vi "AutoDrive.vi"(9 "Target Robot Angle":dbl=-25.0, 10 "Distance":dbl=2000.0, 11 "Movement Angle":dbl) -> (1 "Done":bool=TRUE)   [LabVIEW 2017]
uses:
  Robot Global Data.vi
  <vilib>/addons/control/pid/pid.llb/PID (DBL).vi
  <vilib>/addons/control/pid/NI_PID_pid.lvlib
panel:
  in  "Allowable Encoder Error":dbl=425.0
  out "Encoder Out":dbl=1958.5
  out "output":dbl=0.037765 format="%.2f"
  out "output array":bool[](array[boolean])=[TRUE, TRUE, TRUE, TRUE, TRUE, TRUE, TRUE, TRUE, TRUE, TRUE]
  out "Encoder":cluster{"Robot Angle":dbl, "Gyro":dbl}(graph)={"Robot Angle"=0.0, "Gyro"=-25.0}
  in  "Encoder":dbl
  out "output - Distance":dbl(graph)=1958.5
  out "output - Angle":dbl(graph)=0.09727615381261338
  in  "PID gains - Distance":T1={"proportional gain (Kc)"=0.00091, "integral time (Ti, min)"=0.0, "derivative time (Td, min)"=4.999999999999982e-05} {"derivative time (Td, min)" step=0.001 format="%.5f"; "integral time (Ti, min)" step=0.001 format="%.5f"; "proportional gain (Kc)" step=0.001 format="%.5f"}
  in  "PID gains - Angle":T1={"proportional gain (Kc)"=0.0045, "integral time (Ti, min)"=0.0, "derivative time (Td, min)"=0.0002} {"derivative time (Td, min)" step=0.001 format="%.5f"; "integral time (Ti, min)" step=0.001 format="%.5f"; "proportional gain (Kc)" step=0.001 format="%.5f"}
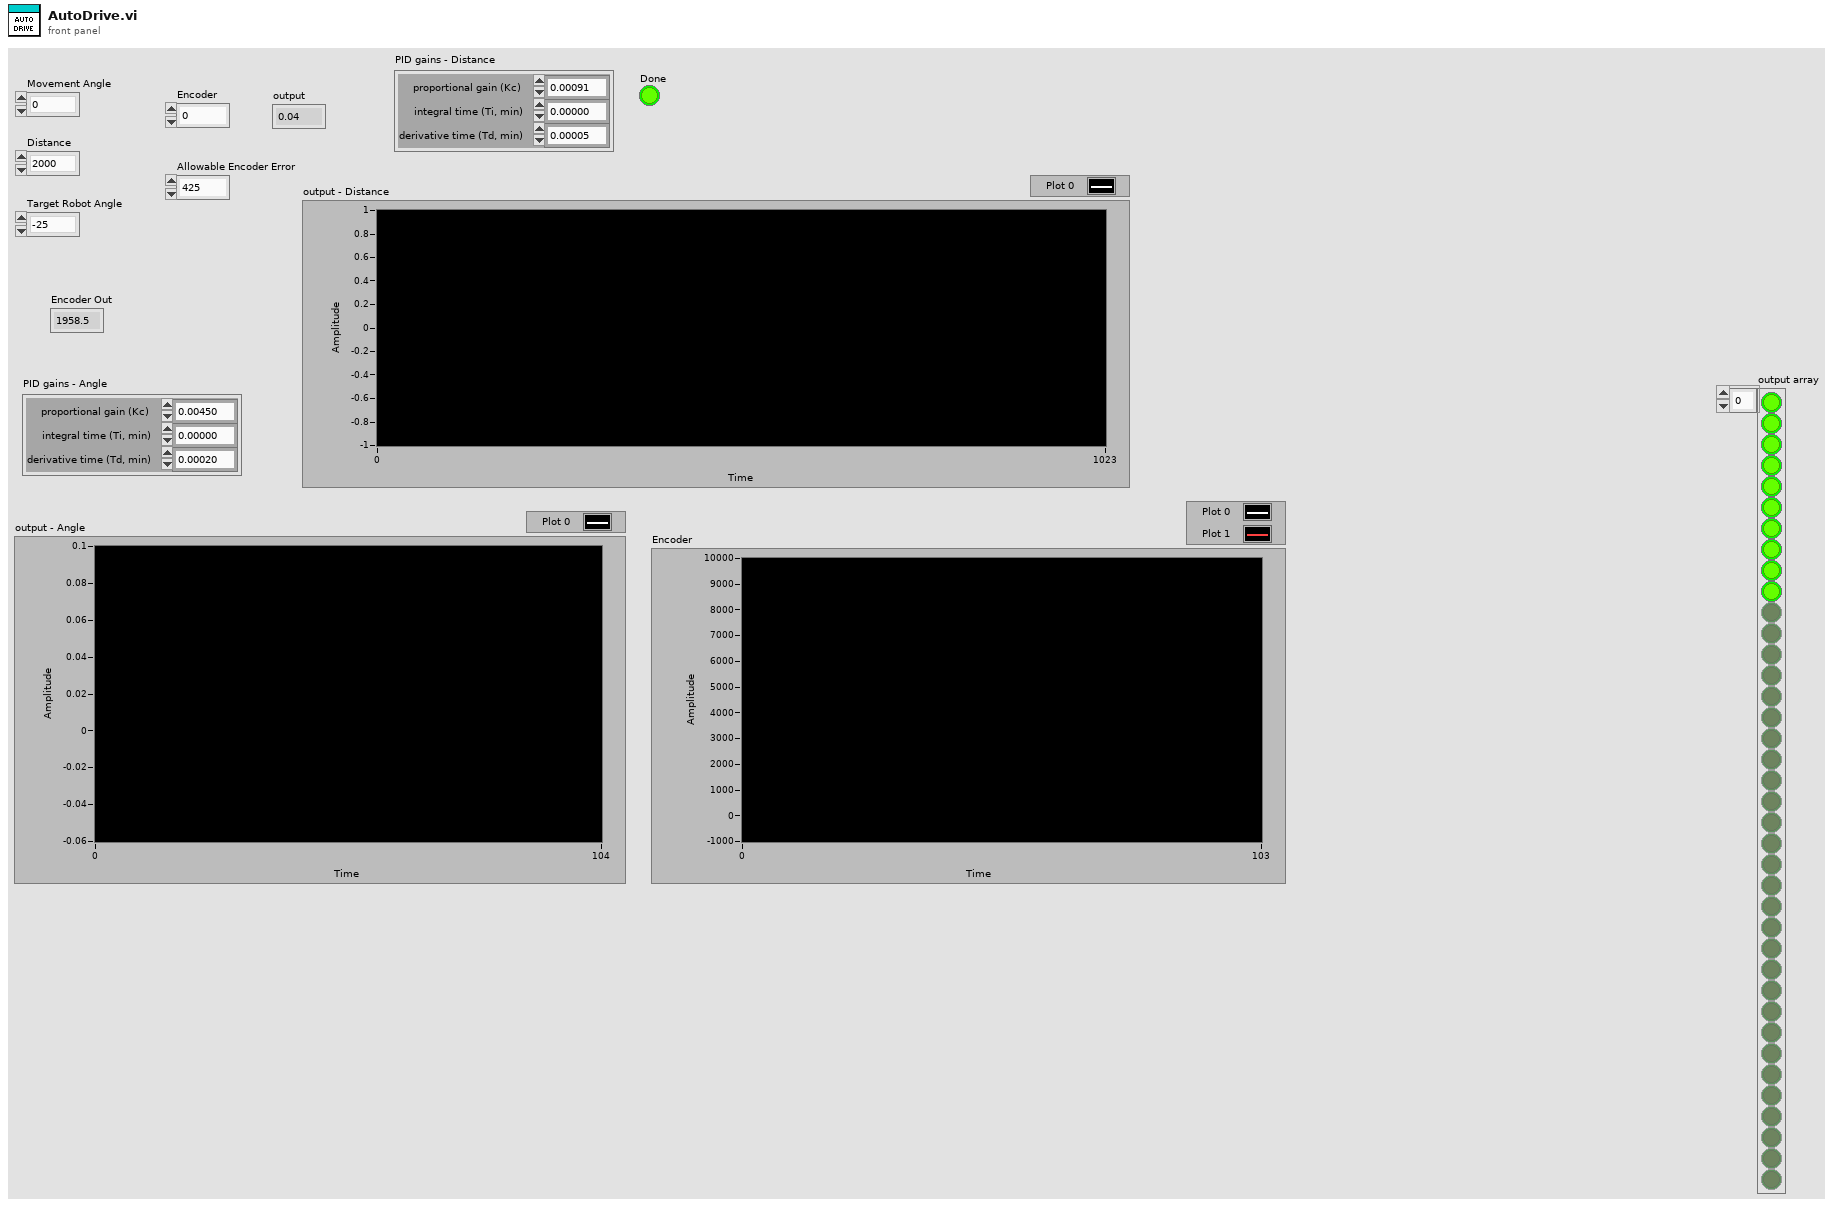
[diagram p1: front panel]
types:
  T1 = cluster{"proportional gain (Kc)":dbl, "integral time (Ti, min)":dbl, "derivative time (Td, min)":dbl}
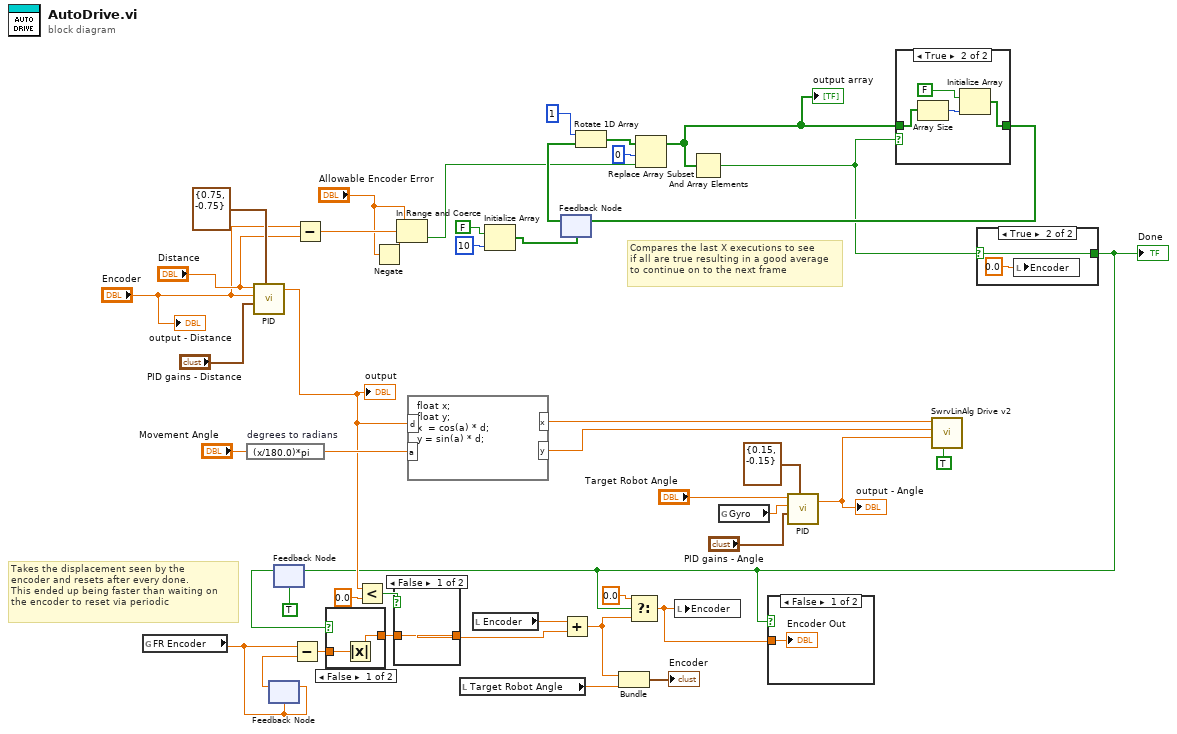
[diagram p0: block diagram]
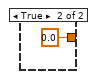
[diagram p2: hidden frame]
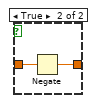
[diagram p5: hidden frame]
diagram:
  # "Compares the last X executions to see\nif all are true resulting in a good average\nto continue on to the next frame"
  # "Takes the displacement seen by the\nencoder and resets after every done.\nThis ended up being faster than waiting on\nthe encoder to reset via periodic"
  n1 = global read "Robot Global Data.vi" "FR Encoder"() -> (w4:dbl)
  n2 = expression code="(x/180.0)*pi" "degrees to radians"("Movement Angle") -> (w20:dbl)
  n3 = call-poly <vilib>:"PID.vi"("output range"=cluster{"output high":dbl, "output low":dbl} {"output high"=0.75, "output low"=-0.75}, "PID gains"="PID gains - Distance", "process variable"="Encoder", "setpoint"="Distance") -> ("output"=w7:dbl)  [unwired: 6 in, 1 out]
  "output" <- w7
  n4 = feedback-in #1(w4) -> ()
  n5 = feedback #1(w4) -> (w5:dbl)
  n6 = feedback #2(TRUE) -> (w3:bool)
  n7 = Subtract(x=w4, y=w5) -> (x-y=w37:dbl)
  n8 = Subtract(x="Encoder", y="Distance") -> (x-y=w11:dbl)
  n9 = case shown="False" w3 {
    tunnel: w37 -> [w47 _]
    tunnel: [w46 0.0] -> w34
    frame False {
      n10 = Absolute Value(x=w47) -> (abs(x)=w46:dbl)
    }
    frame True {
    }
  }
  n11 = Less?(x=w7, y=0.0) -> (x < y?=w35:bool)
  n12 = Negate(x="Allowable Encoder Error") -> (-x=w38:dbl)
  n13 = case shown="False" w35 {
    tunnel: w34 -> [w49 w51]
    tunnel: [w49 w50] -> w17
    frame False {
    }
    frame True {
      n14 = Negate(x=w51) -> (-x=w50:dbl)
    }
  }
  n15 = In Range and Coerce(upper limit="Allowable Encoder Error", x=w11, lower limit=w38) -> (In Range?=w21:bool)  [unwired: 1 out]
  n16 = formula code="float x;\nfloat y;\nx  = cos(a) * d;\ny = sin(a) * d;"("d"=w7, "a"=w20) -> ("x"=w18:dbl, "y"=w19:dbl)
  n17 = local read "Target Robot Angle"() -> (w14:dbl)
  n18 = local read "Encoder"() -> (w32:dbl)
  n19 = Initialize Array(FALSE, 10 ("dimension size")) -> (w24:bool[])
  n20 = feedback #3(w24) -> (w27:bool[])
  n21 = Add(x=w32, y=w17) -> (x+y=w33:dbl)
  n22 = Rotate 1D Array(1:w27, 2:1 ("n")) -> (0:w29:bool[])
  n23 = Bundle(w33, "Target Robot Angle"=w14) -> (→"Encoder":cluster{dbl, "Target Robot Angle":dbl})  [unwired: 1 in]
  n24 = Replace Array Subset(array=w29, new element=w21, index=0) -> (w25:bool[])
  "output array" <- w25
  n25 = And Array Elements(Boolean array=w25) -> (logical AND=w6:bool)
  n26 = global read "Robot Global Data.vi" "Gyro"() -> (w39:dbl)
  n27 = call-poly <vilib>:"PID.vi"("output range"=cluster{"output high":dbl, "output low":dbl} {"output high"=0.15, "output low"=-0.15}, "PID gains"="PID gains - Angle", "process variable"=w39, "setpoint"="Target Robot Angle") -> ("output"=w8:dbl)  [unwired: 6 in, 1 out]
  "output - Angle" <- w8
  n28 = case shown="True" w6 {
    tunnel: w25 -> [w52 w54]
    tunnel: [w52 w53] -> w26
    frame False {
    }
    frame True {
      n29 = Array Size(array=w54) -> (size(s)=w55:i32)
      n30 = Initialize Array(FALSE, w55) -> (w53:bool[])
    }
  }
  n31 = feedback-in #3(w26) -> ()
  n32 = call "SwrvLinAlg Drive v2.vi"("Auto Controls"=TRUE, "Z"=w8, "Y"=w19, "X"=w18) -> ()  [unwired: 8 in]
  n33 = case shown="True" w6 {
    selector: w6 -> [w57 w58]
    tunnel: [w57 w58] -> w2
    frame False {
    }
    frame True {
      n34 = local write "Encoder"(0.0 ("Encoder")) -> ()
    }
  }
  "Done" <- w2
  n35 = feedback-in #2(w2) -> ()
  n36 = Select(t=0.0, s=w2, f=w33) -> (s? t:f=w13:dbl)
  n37 = local write "Encoder"(w13) -> ()
  n38 = case shown="False" w2 {
    tunnel: w13 -> [w60 _]
    frame False {
      "Encoder Out" <- w60
    }
    frame True {
    }
  }
  "output - Distance" <- "Encoder"
